vi "Image Processing Main test bench.vi"() -> ()   [LabVIEW 2009]
panel:
  out "Ramp?":bool
  out "left 2":T1(plugin-control)
  out "right 2":T1(plugin-control)
  out "Waveform Graph":u16[](graph)
  out "Image Type":T2 items=["Grayscale (U8)", "Grayscale (I16)", "Grayscale (SGL)", "Complex (CSG)", "RGB (U32)", "HSL (U32)", "RGB (U64)", "Grayscale (U16)"]
  out "left":T1(plugin-control)
  in  "File Path L":path
  out "right":T1(plugin-control)
  in  "File Path R":path
  in  "Extraction mode":i32(knob) scale=0.0..2.0
  out "Number of ramp regions (left)":i32
  out "Number of ramp regions (right)":i32
  out "Sick array":u16[](array[numeric])
  # "0: Old line extraction\n1: Solid white line (ramp)\n2: LPF"
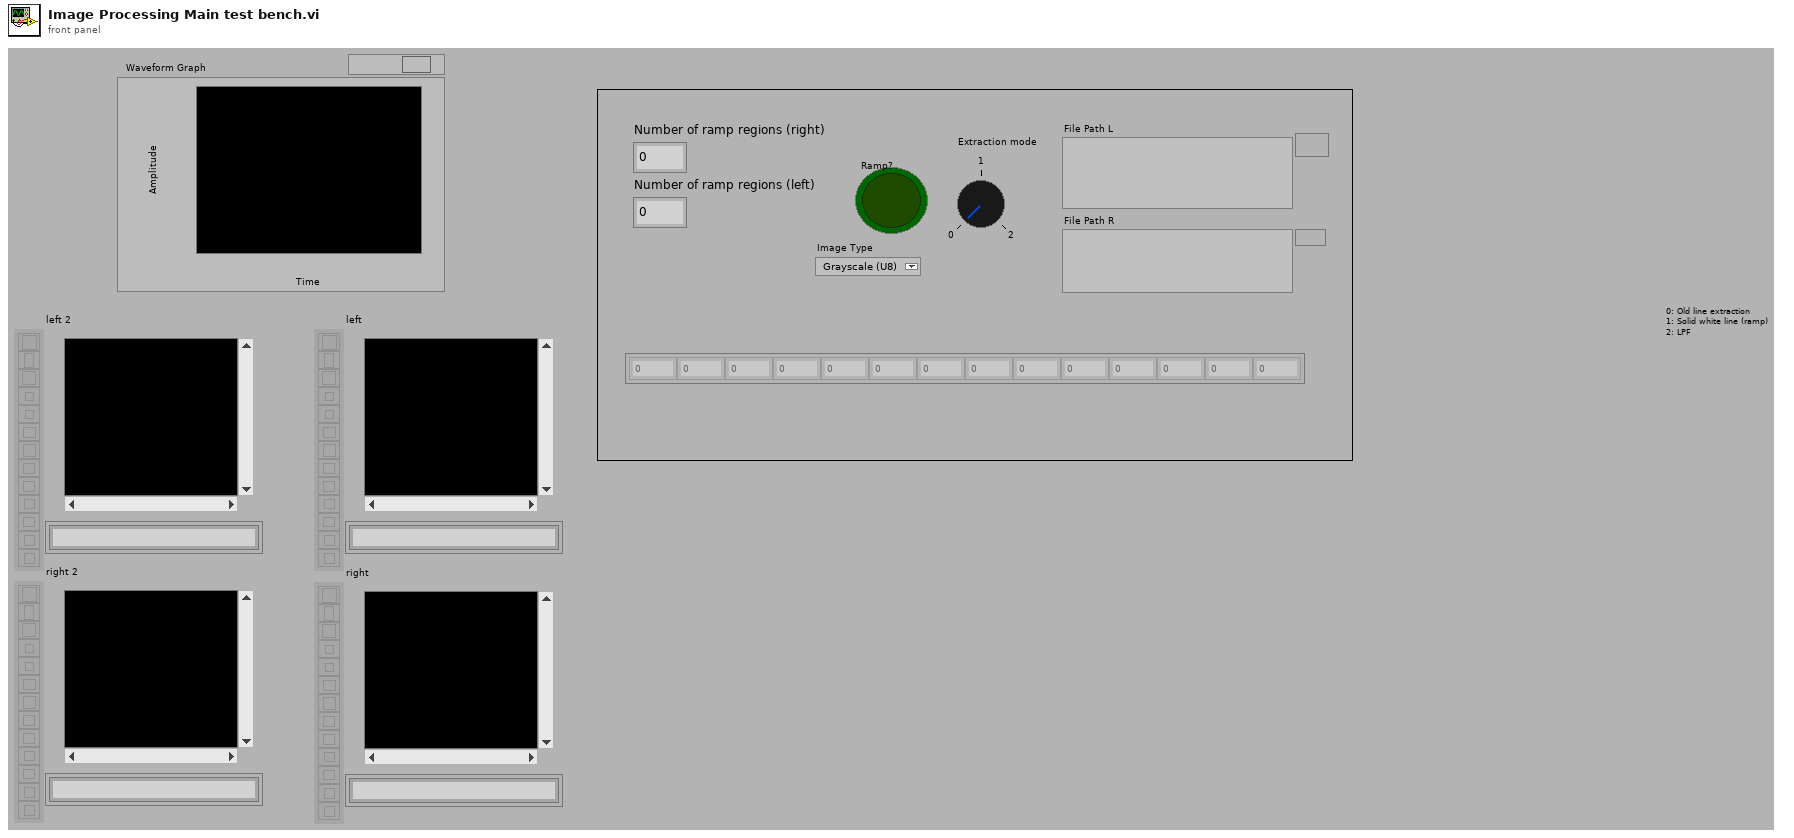
[diagram p1: front panel]
types:
  T1 = typedef "IMAQ Image.ctl" = refnum<image>
  T2 = typedef "Image Type" = u32
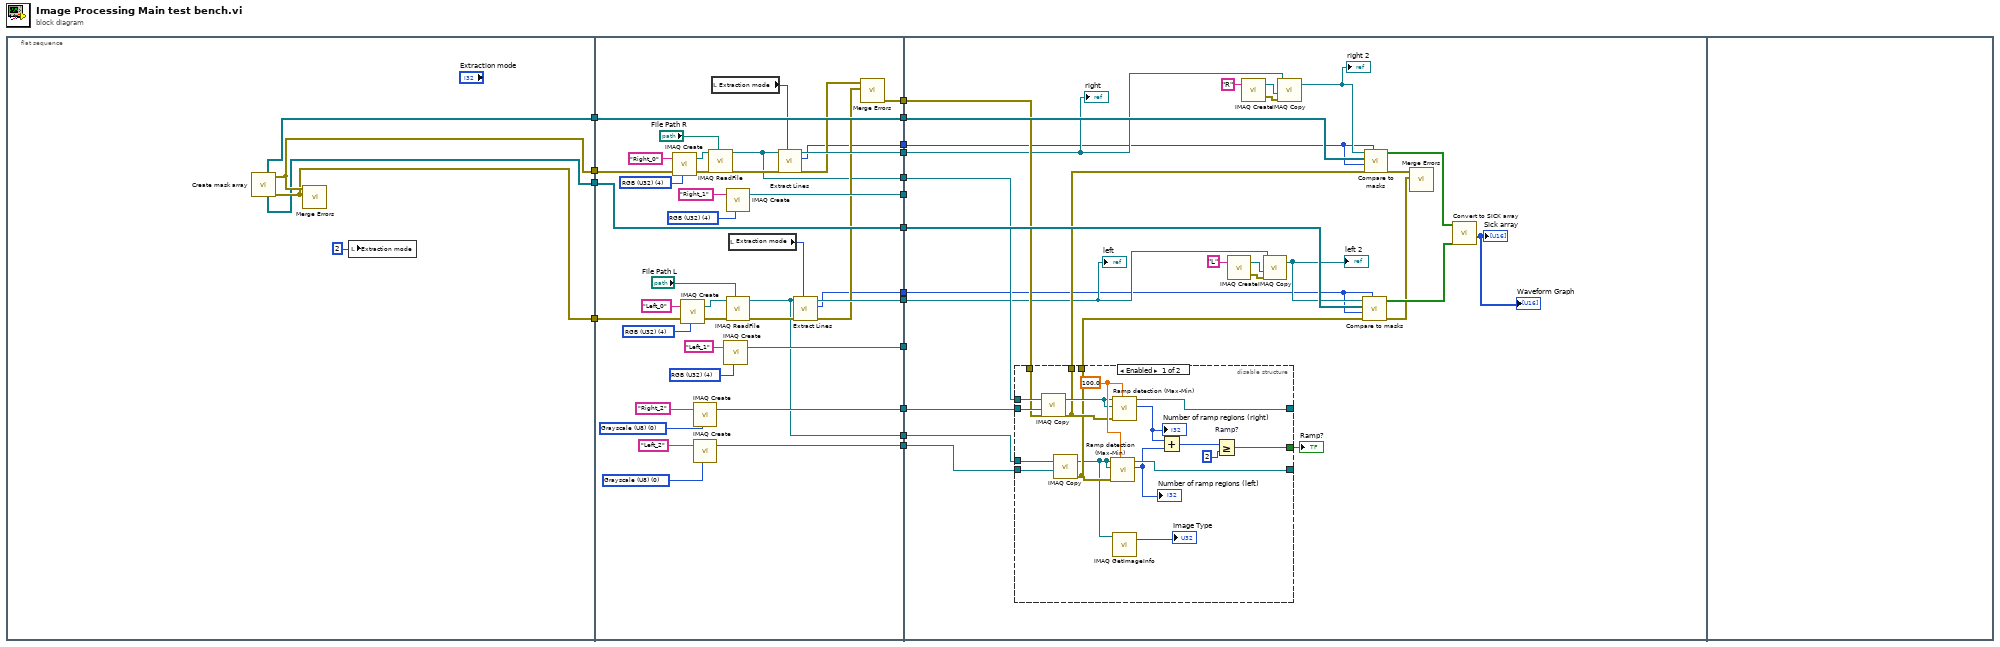
[diagram p0: block diagram]
diagram:
  n1 = flat-sequence {
    tunnel: [w22] -> w17
    tunnel: [w21] -> w16
    tunnel: [w20] -> w11
    tunnel: [w19] -> w10
    tunnel: w17 -> [w61]
    tunnel: w16 -> [w60]
    tunnel: [w57] -> w15
    tunnel: [w54] -> w14
    tunnel: [w53] -> w13
    tunnel: [w52] -> w12
    tunnel: w11 -> [w51]
    tunnel: w10 -> [w50]
    tunnel: [w51] -> w9
    tunnel: [w50] -> w8
    tunnel: [w47] -> w7
    tunnel: [w46] -> w6
    tunnel: [w43] -> w5
    tunnel: [w26] -> w4
    tunnel: [w25] -> w3
    tunnel: [w24] -> w2
    tunnel: [w23] -> w1
    tunnel: w15 -> [_]
    tunnel: w14 -> [_]
    tunnel: w13 -> [w71]
    tunnel: w12 -> [w67]
    tunnel: w9 -> [w88]
    tunnel: w8 -> [w87]
    tunnel: w7 -> [w86]
    tunnel: w6 -> [w85]
    tunnel: w5 -> [w80]
    tunnel: w4 -> [w77]
    tunnel: w3 -> [w76]
    tunnel: w2 -> [w64]
    tunnel: w1 -> [w63]
    frame #0 {
      n2 = call "Create mask array.vi"() -> ("Left error out"=w21:errorcluster, "Right error out"=w22:errorcluster, "Left Cam Masks"=w19:T1[], "Right Cam Masks"=w20:T1[])  [unwired: 8 in]
      n3 = call <vilib>:"Merge Errors.vi"("error in 2 (no error)"=w21, "error in 1 (no error)"=w22) -> ()  [unwired: 5 in, 1 out]
      n4 = local write "Extraction mode"(2 ("Extraction mode")) -> ()
    }
    frame #1 {
      w27 = T2 4 items=["Grayscale (U8)", "Grayscale (I16)", "Grayscale (SGL)", "Complex (CSG)", "RGB (U32)", "HSL (U32)", "RGB (U64)", "Grayscale (U16)"] ("Image Type")
      w28 = T2 4 items=["Grayscale (U8)", "Grayscale (I16)", "Grayscale (SGL)", "Complex (CSG)", "RGB (U32)", "HSL (U32)", "RGB (U64)", "Grayscale (U16)"] ("Image Type")
      w29 = T2 4 items=["Grayscale (U8)", "Grayscale (I16)", "Grayscale (SGL)", "Complex (CSG)", "RGB (U32)", "HSL (U32)", "RGB (U64)", "Grayscale (U16)"] ("Image Type")
      w30 = T2 4 items=["Grayscale (U8)", "Grayscale (I16)", "Grayscale (SGL)", "Complex (CSG)", "RGB (U32)", "HSL (U32)", "RGB (U64)", "Grayscale (U16)"] ("Image Type")
      w41 = T2 0 items=["Grayscale (U8)", "Grayscale (I16)", "Grayscale (SGL)", "Complex (CSG)", "RGB (U32)", "HSL (U32)", "RGB (U64)", "Grayscale (U16)"] ("Image Type")
      w42 = T2 0 items=["Grayscale (U8)", "Grayscale (I16)", "Grayscale (SGL)", "Complex (CSG)", "RGB (U32)", "HSL (U32)", "RGB (U64)", "Grayscale (U16)"] ("Image Type")
      n5 = call "IMAQ Create"("Image Name"="Right_0", "Image Type"=w30, "error in (no error)"=w61) -> ("New Image"=w40:T1, "error out"=w39:errorcluster)  [unwired: 2 in]
      n6 = call "IMAQ Create"("Image Name"="Left_0", "Image Type"=w28, "error in (no error)"=w60) -> ("New Image"=w36:T1, "error out"=w35:errorcluster)  [unwired: 2 in]
      n7 = call "IMAQ Create"("Image Name"="Right_2", "Image Type"=w42) -> ("New Image"=w47:T1)  [unwired: 3 in, 1 out]
      n8 = call "IMAQ Create"("Image Name"="Left_2", "Image Type"=w41) -> ("New Image"=w46:T1)  [unwired: 3 in, 1 out]
      n9 = call "IMAQ ReadFile"("File Path"="File Path R", "error in (no error)"=w39, "Image"=w40) -> ("error out"=w38:errorcluster, "Image Out"=w26:T1)  [unwired: 4 in, 3 out]
      n10 = local read "Extraction mode"() -> (w34:i32)
      n11 = call "IMAQ Create"("Image Name"="Left_1", "Image Type"=w27) -> ("New Image"=w54:T1)  [unwired: 3 in, 1 out]
      n12 = call "IMAQ Create"("Image Name"="Right_1", "Image Type"=w29) -> ("New Image"=w57:T1)  [unwired: 3 in, 1 out]
      n13 = call "IMAQ ReadFile"("File Path"="File Path L", "error in (no error)"=w35, "Image"=w36) -> ("error out"=w37:errorcluster, "Image Out"=w25:T1)  [unwired: 4 in, 3 out]
      n14 = local read "Extraction mode"() -> (w33:i32)
      n15 = call "Extract Lines.vi"("Extraction mode"=w34, "error in (no error)"=w38, "Image Src"=w26) -> ("error out"=w45:errorcluster, "Number of Particles1"=w24:i32, "Image Out"=w53:T1)  [unwired: 6 in]
      n16 = call "Extract Lines.vi"("Extraction mode"=w33, "error in (no error)"=w37, "Image Src"=w25) -> ("error out"=w44:errorcluster, "Number of Particles1"=w23:i32, "Image Out"=w52:T1)  [unwired: 6 in]
      n17 = call <vilib>:"Merge Errors.vi"("error in 2 (no error)"=w44, "error in 1 (no error)"=w45) -> ("error out"=w43:errorcluster)  [unwired: 5 in]
    }
    frame #2 {
      n18 = disable-structure shown="Enabled" {
        disable-tunnel: [w106 _] -> _
        disable-tunnel: [w105 _] -> _
        disable-tunnel: [w99 _] -> w62
        disable-tunnel: w86 -> [w98 _]
        disable-tunnel: w85 -> [w97 _]
        disable-tunnel: [w95 _] -> w79
        disable-tunnel: [w94 _] -> w78
        disable-tunnel: w77 -> [w93 _]
        disable-tunnel: w76 -> [w92 _]
        disable-tunnel: w80 -> [w91 _]
        frame #0 {
          w104 = sgl 100.0 ("Tolerance")
          n19 = call "IMAQ Copy"("error in (no error)"=w91, "Image Dst"=w98, "Image Src"=w93) -> ("error out"=w95:errorcluster, "Image Dst Out"=w96:T1)  [unwired: 3 in]
          n20 = call "IMAQ Copy"("Image Dst"=w97, "Image Src"=w92) -> ("error out"=w94:errorcluster, "Image Dst Out"=w90:T1)  [unwired: 4 in]
          n21 = call "Ramp detection (Max-Min).vi"("Tolerance"=w104, "error in (no error)"=w94, "Image Dst"=w90, "Image Src"=w90) -> ("Number of ramp regions"=w102:i32, "Image Out"=w105:T1)  [unwired: 5 in, 1 out]
          "Number of ramp regions (left)" <- w102
          n22 = call "Ramp detection (Max-Min).vi"("Tolerance"=w104, "error in (no error)"=w95, "Image Dst"=w96, "Image Src"=w96) -> ("Number of ramp regions"=w103:i32, "Image Out"=w106:T1)  [unwired: 5 in, 1 out]
          "Number of ramp regions (right)" <- w103
          n23 = call "IMAQ GetImageInfo"("Image"=w90) -> ("Image Type"=→"Image Type":T2)  [unwired: 3 in, 7 out]
          n24 = Add(x=w103, y=w102) -> (x+y=w101:i32)
          n25 = Greater Or Equal? "Ramp?"(x=w101, y=2) -> (x >= y?=w99:bool)
        }
        frame #1 {
        }
      }
      "Ramp?" <- w62
      n26 = call "IMAQ Create"("Image Name"="L") -> ("New Image"=w70:T1, "error out"=w68:errorcluster)  [unwired: 4 in]
      n27 = call "IMAQ Create"("Image Name"="R") -> ("New Image"=w72:T1, "error out"=w74:errorcluster)  [unwired: 4 in]
      n28 = call "IMAQ Copy"("error in (no error)"=w68, "Image Dst"=w70, "Image Src"=w67) -> ("Image Dst Out"=w65:T1)  [unwired: 3 in, 1 out]
      "left 2" <- w65
      n29 = call "IMAQ Copy"("error in (no error)"=w74, "Image Dst"=w72, "Image Src"=w71) -> ("Image Dst Out"=w66:T1)  [unwired: 3 in, 1 out]
      "right 2" <- w66
      n30 = call "Compare to masks.vi"("Number of Particles1"=w63, "error in (no error)"=w78, "Number of Particles"=w63, "Mask array"=w87, "Image Src"=w65) -> ("Final error out"=w81:errorcluster, "Marked Regions"=w83:bool[])  [unwired: 5 in]
      n31 = call "Compare to masks.vi"("Number of Particles1"=w64, "error in (no error)"=w79, "Number of Particles"=w64, "Mask array"=w88, "Image Src"=w66) -> ("Final error out"=w82:errorcluster, "Marked Regions"=w84:bool[])  [unwired: 5 in]
      n32 = call <vilib>:"Merge Errors.vi"("error in 2 (no error)"=w81, "error in 1 (no error)"=w82) -> ()  [unwired: 5 in, 1 out]
      n33 = call "Convert to SICK array.vi"("Left Regions"=w83, "Right Regions"=w84) -> ("Sick array"=→"Sick array" →"Waveform Graph":u16[])  [unwired: 9 in]
      "right" <- w71
      "left" <- w67
    }
    frame #3 {
    }
  }
